vi "ImageConnection_Multiple.vi"(1 "Image Name":string, 2 "Image Subscriber list":string, 3 "Nr.":i32) -> ()   [LabVIEW 2013]
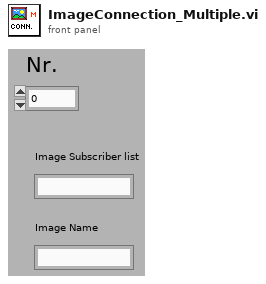
[diagram p1: front panel]
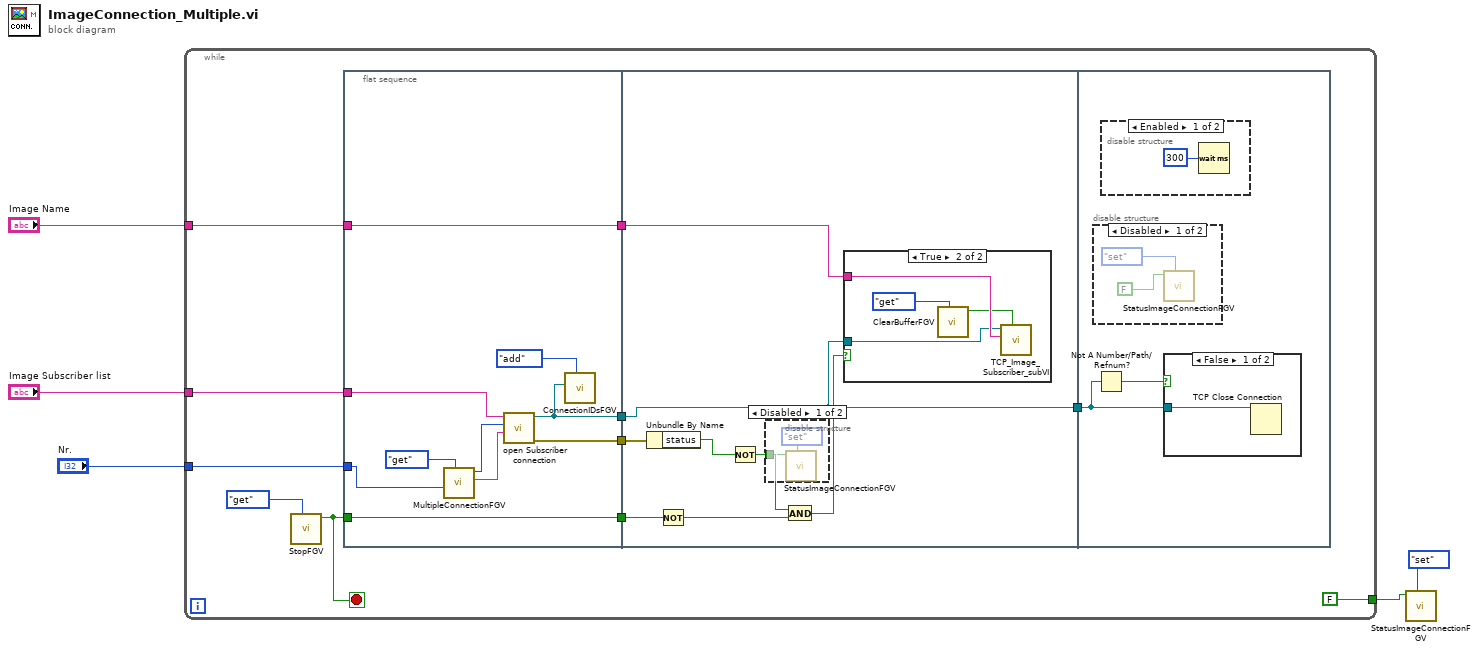
[diagram p0: block diagram]
diagram:
  n1 = while {
    tunnel: "Image Name" -> [w16]
    tunnel: "Image Subscriber list" -> [w15]
    tunnel: [FALSE] -> w2
    tunnel: "Nr." -> [w6]
    stop <- w12 stop-if-true
    n2 = call "StopFGV.vi"("Command"=enum16{"set", "get", "init"}."get") -> ("Stop out"=w12:bool)  [unwired: 9 in, 1 out]
    n3 = flat-sequence {
      tunnel: w16 -> [w22]
      tunnel: [w22] -> w11
      tunnel: w15 -> [w26]
      tunnel: w12 -> [w21]
      tunnel: [w21] -> w10
      tunnel: [w23] -> w9
      tunnel: [w25] -> w8
      tunnel: w6 -> [w19]
      tunnel: w11 -> [w34]
      tunnel: w10 -> [w30]
      tunnel: w9 -> [w33]
      tunnel: [w33] -> w7
      tunnel: w8 -> [w32]
      tunnel: w7 -> [w41]
      frame #0 {
        n4 = call "MultipleConnectionFGV.vi"("command"=enum16{"get", "set", "init"}."get", "Nr."=w19) -> ("Remote Host out"=w17:string, "port or service name out"=w18:u16)  [unwired: 8 in]
        n5 = call "open Subscriber connection.vi"("Machine"=w17, "Port"=w18, "Subscriber list"=w26) -> ("error out"=w25:errorcluster, "connection ID"=w23:refnum<k5>)  [unwired: 3 in]
        n6 = call "ConnectionIDsFGV.vi"("Command"=enum16{"add", "get", "init"}."add", "connection ID"=w23) -> ()  [unwired: 9 in, 1 out]
      }
      frame #1 {
        n7 = Unbundle By Name(w32) -> ("status"=w31:bool)
        n8 = Not(x=w30) -> (.not. x?=w29:bool)
        n9 = Not(x=w31) -> (.not. x?=w27:bool)
        n10 = disable-structure shown="Disabled" {
          disable-tunnel: w27 -> [w36 _]
          frame Disabled {
            n11 = call "StatusImageConnectionFGV.vi"("Command"=enum16{"get", "set", "init"}."set", "Image Connection"=w36) -> ()  [unwired: 9 in, 1 out]
          }
          frame Enabled {
          }
        }
        n12 = And(x=w27, y=w29) -> (x .and. y?=w28:bool)
        n13 = case shown="True" w28 {
          tunnel: w34 -> [_ w40]
          tunnel: w33 -> [_ w39]
          frame False {
          }
          frame True {
            n14 = call "ClearBufferFGV.vi"("Command"=enum16{"set", "get", "init"}."get") -> ("clear buffer out"=w37:bool)  [unwired: 10 in]
            n15 = call "TCP_Image_Subscriber_subVI.vi"("clear buffer"=w37, "Image Name"=w40, "connection ID"=w39) -> ()  [unwired: 8 in, 1 out]
          }
        }
      }
      frame #2 {
        n16 = disable-structure shown="Disabled" {
          frame Disabled {
            n17 = call "StatusImageConnectionFGV.vi"("Command"=enum16{"get", "set", "init"}."set", "Image Connection"=FALSE ("status")) -> ()  [unwired: 9 in, 1 out]
          }
          frame Enabled {
          }
        }
        n18 = Not A Number/Path/Refnum?(number/path/refnum=w41) -> (NaN/Path/Refnum?=w42:bool)
        n19 = disable-structure shown="Enabled" {
          frame Enabled {
            n20 = Wait (ms)(milliseconds to wait=u32 300 ("millisecond multiple")) -> ()  [unwired: 1 out]
          }
          frame Disabled {
          }
        }
        n21 = case shown="False" w42 {
          tunnel: w41 -> [w46 _]
          frame False {
            n22 = TCP Close Connection(connection ID=w46) -> ()  [unwired: 2 in, 2 out]
          }
          frame True {
          }
        }
      }
    }
  }
  n23 = call "StatusImageConnectionFGV.vi"("Command"=enum16{"get", "set", "init"}."set", "Image Connection"=w2) -> ()  [unwired: 9 in, 1 out]
